vi "DDC (Single Channel, IQ Power Trigger).vi"(0 "data in":T4, 1 "reset":bool, 5 "start trigger":bool, 7 "power level trigger configuration":T1 {"trig level" format="%#.48g"}, 9 "enabled":bool, 11 "DDC Parameters":T2={"output sample rate"=1.0, "delay"=0.0, "frequency shift"=0.0, "impairments"={"inline gain I"=0.9999923706054688, "inline gain Q"=0.9999923706054688, "cross gain I"=0.0, "cross gain Q"=0.0, "pre-gain offset I"=0.0, "pre-gain offset Q"=0.0, "post-gain offset I"=0.0, "post-gain offset Q"=0.0}, "phase"=0.0} {"frequency shift" format="%#.48g"}, 13 "ready for trigger":bool=TRUE) -> (4 "data out":u32, 6 "number of overflows":u64, 8 "power level trigger":bool, 10 "output valid":bool, 14 "dsp reset done":bool)   [LabVIEW 2015]
doc: "Controls whether or not data is written to the DMA FIFO for the acquisition stream. If burst size is 0, this will be a continuous stream, started when the start trigger is asserted. If burst size is greater than zero, acquisition will be in bursts of the designated size, initiated each time the internal state machine is idle and a start trigger is received.\n\nThis VI also keeps track of whether or not an overflow occurred in the acquisition stream and counts the number of overflows that have occurred for debugging information.\n\nThe internal state machine returns the number of samples processed since the most recent acquisition began and the current state machine state."
uses:
  <instrlib>/_niInstr/DSP/v1/Shared/Public/IQ Data.ctl
  DDC Parameters.ctl
  <instrlib>/_niInstr/DSP/v1/Shared/Public/IQ Impairments.ctl
  <instrlib>/_niInstr/DSP/v1/Shared/Public/IQ Power Level Configuration - 36 bit.ctl
  <instrlib>/_niInstr/Basic Elements/v1/FPGA/Private/Count Up U64.vi
  <instrlib>/_niInstr/DSP/v1/FPGA/Public/Sub VIs/IQ Impairments/IQ Impairments - 1 spc.vi
  <instrlib>/_niInstr/DSP/v1/FPGA/Public/Sub VIs/Frequency Shift/Frequency Shift - 1 spc.vi
  <instrlib>/_niInstr/DSP/v1/FPGA/Public/Sub VIs/Fractional Decimator/Fractional Decimator - 1 spc - 2x oc.vi
  <instrlib>/_niInstr/DSP/v1/FPGA/Public/Sub VIs/IQ Power Level Trigger/IQ Power Level Trigger - 1 spc - 18 bit.vi
  <instrlib>/_niInstr/DSP/v1/FPGA/niInstr DSP v1 FPGA.lvlib
  <instrlib>/_niInstr/Basic Elements/v1/FPGA/niInstr Basic Elements v1 FPGA.lvlib
  <instrlib>/_niInstr/DSP/v1/Shared/niInstr DSP v1 Shared.lvlib
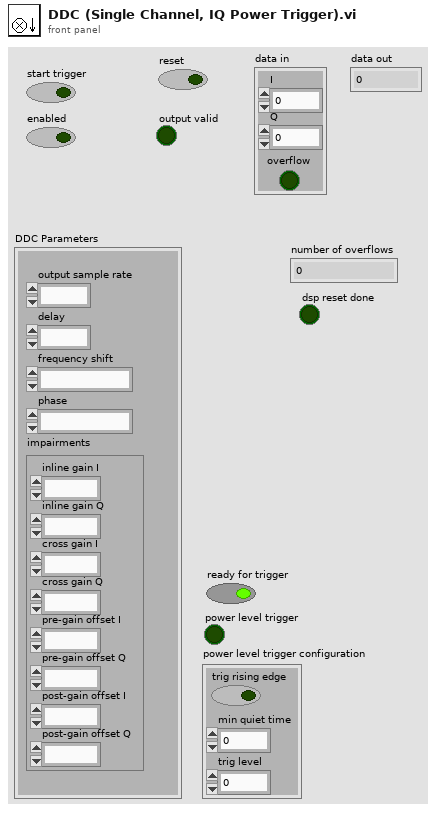
[diagram p1: front panel]
types:
  T1 = typedef "niInstr DSP v1 Shared.lvlib/IQ Power Level Configuration - 36 bit.ctl" = cluster{"trig rising edge":bool, "min quiet time":u32, "trig level":fxp<+,36,2>}
  T2 = typedef "DDC Parameters.ctl" = cluster{"output sample rate":fxp<+,48,1>, "delay":fxp<+/-,16,0>, "frequency shift":fxp<+/-,48,0>, "impairments":T3, "phase":fxp<+/-,21,0>}
  T3 = typedef "niInstr DSP v1 Shared.lvlib/IQ Impairments.ctl" = cluster{"inline gain I":fxp<+/-,18,1>, "inline gain Q":fxp<+/-,18,1>, "cross gain I":fxp<+/-,18,1>, "cross gain Q":fxp<+/-,18,1>, "pre-gain offset I":fxp<+/-,18,1>, "pre-gain offset Q":fxp<+/-,18,1>, "post-gain offset I":fxp<+/-,18,1>, "post-gain offset Q":fxp<+/-,18,1>}
  T4 = typedef "niInstr DSP v1 Shared.lvlib/IQ Data.ctl" = cluster{"I":fxp<+/-,18,1>, "Q":fxp<+/-,18,1>, "overflow":bool}
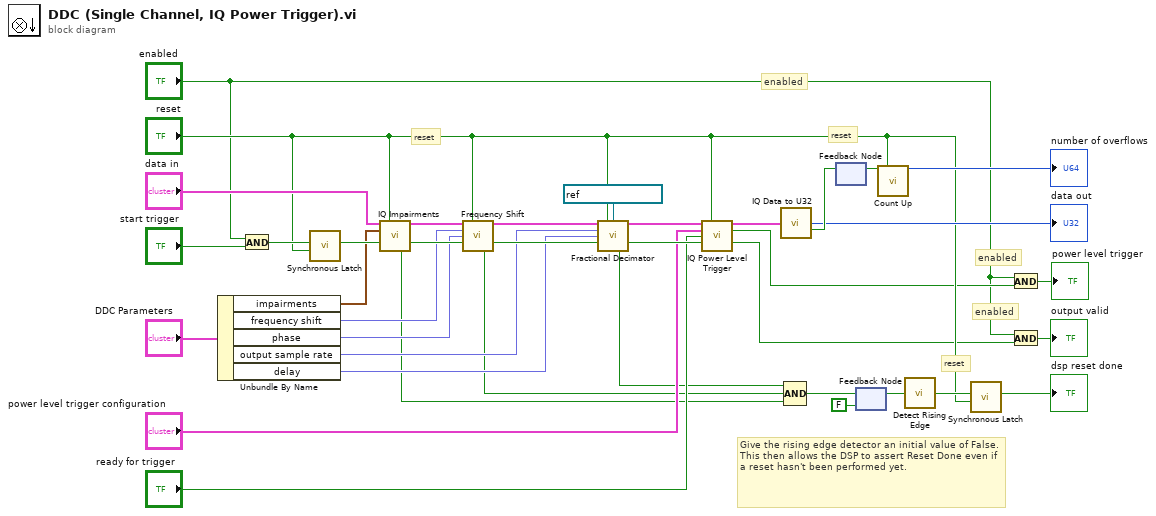
[diagram p0: block diagram]
diagram:
  # "enabled"
  # "Give the rising edge detector an initial value of False.  This then allows the DSP to assert Reset Done even if a reset hasn't been performed yet."
  # "reset"
  # "reset"
  # "reset"
  # "enabled"
  # "enabled"
  n1 = Unbundle By Name("DDC Parameters") -> ("impairments"=w32:T3, "frequency shift"=w31:fxp<+/-,48,0>, "phase"=w30:fxp<+/-,21,0>, "output sample rate"=w29:fxp<+,48,1>, "delay"=w28:fxp<+/-,16,0>)
  n2 = And(x="enabled", y="start trigger") -> (x .and. y?=w25:bool)
  n3 = call <instrlib>:"Synchronous Latch.vi"("clear"="reset", "set"=w25) -> ("out"=w36:bool)  [unwired: 9 in]
  n4 = call-poly <instrlib>:"IQ Impairments.vi"("data in"="data in", "reset"="reset", "impairments"=w32, "input valid"=w36) -> ("data out"=w37:T4, "output valid"=w35:bool, "ready for input"=w1:bool)  [unwired: 9 in]
  n5 = call-poly <instrlib>:"Frequency Shift.vi"("data in"=w37, "reset"="reset", "frequency shift"=w31, "phase"=w30, "input valid"=w35) -> ("data out"=w38:T4, "output valid"=w34:bool, "ready for input"=w2:bool)  [unwired: 8 in]
  n6 = call-poly <instrlib>:"Fractional Decimator.vi"("data in"=w38, "reset"="reset", "clock x 2"=refnum<k21> "Data Clock x2" ("oversample clock"), "output sample rate"=w29, "delay"=w28, "input valid"=w34) -> ("data out"=w14:T4, "output valid"=w10:bool, "ready for input"=w3:bool)  [unwired: 7 in]
  n7 = call-poly <instrlib>:"IQ Power Level Trigger.vi"("input data"=w14, "reset"="reset", "configuration"="power level trigger configuration", "ready for trigger"="ready for trigger", "input valid"=w10) -> ("output data"=w13:T4, "trigger"=w7:bool, "output valid"=w11:bool)  [unwired: 8 in]
  n8 = call <instrlib>:"IQ Data to U32.vi"("IQ data"=w13) -> ("U32 data"=→"data out":u32, "overflow"=w22:bool)  [unwired: 13 in]
  n9 = Compound Arithmetic op=AND(w3, w2, w1) -> (w4:bool)
  n10 = feedback #1() -> (w21:bool)  [unwired: 1 in]
  n11 = feedback-in #1(w22) -> ()
  n12 = feedback-in #2(w4) -> ()
  n13 = feedback #2(FALSE ("ready for input")) -> (w16:bool)
  n14 = call-poly <instrlib>:"Count Up.vi"("increment"=w21, "reset"="reset") -> ("count out"=→"number of overflows":u64)  [unwired: 13 in]
  n15 = call <instrlib>:"Detect Rising Edge.vi"("signal"=w16) -> ("edge detected"=w33:bool)  [unwired: 14 in]
  n16 = call <instrlib>:"Synchronous Latch.vi"("clear"="reset", "set"=w33) -> ("out"=→"dsp reset done":bool)  [unwired: 9 in]
  n17 = And(x="enabled", y=w7) -> (x .and. y?=→"power level trigger":bool)
  n18 = And(x="enabled", y=w11) -> (x .and. y?=→"output valid":bool)
